vi "TestWordSearch.vi"   [LabVIEW 2022 SP3]
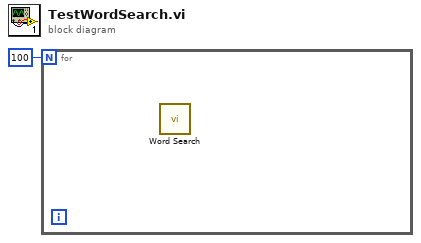
[diagram p0: block diagram]
diagram:
  n1 = for {
    N: 100 -> [_]
    n2 = call "Word Search.vi"() -> ()  [unwired: 12 in]
  }
